vi "Sleep Until Future Time.vi"(7 "FTE Limits (ns)":T1={"Maximum"=200000000, "Minimum"=20000} {"Maximum" format="%.0e"; "Minimum" format="%.0e"}, 8 "error in (no error)":errorcluster, 10 "Wake Time":u64, 11 "ClockID":u16) -> (0 "error out":errorcluster)   [LabVIEW 2021, in "CIFClocks.lvlib"]
uses:
  CIFClocks.lvlib
  Typedef/Future Time Event Limits.ctl
  Typedef/Errors.ctl
  Time Conversion/LabVIEW Time to UTC Time.vi
  CIFCore/CIFCoreCommon/CIFCoreCommon.lvlib
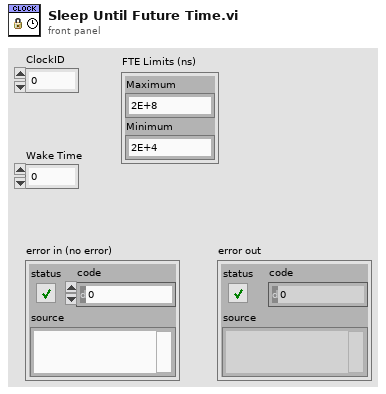
[diagram p1: front panel]
types:
  T1 = typedef "CIFClocks.lvlib/Future Time Event Limits.ctl" = cluster{"Maximum":u64, "Minimum":u64}
  T2 = typedef "CIFCoreCommon.lvlib/Errors.ctl" = enum16{"Invalid Clock ID", "Long Sleep", "gRPC Server Not Found", "Config Parse", "Timestamp Wrap", "Delayed Execution"}
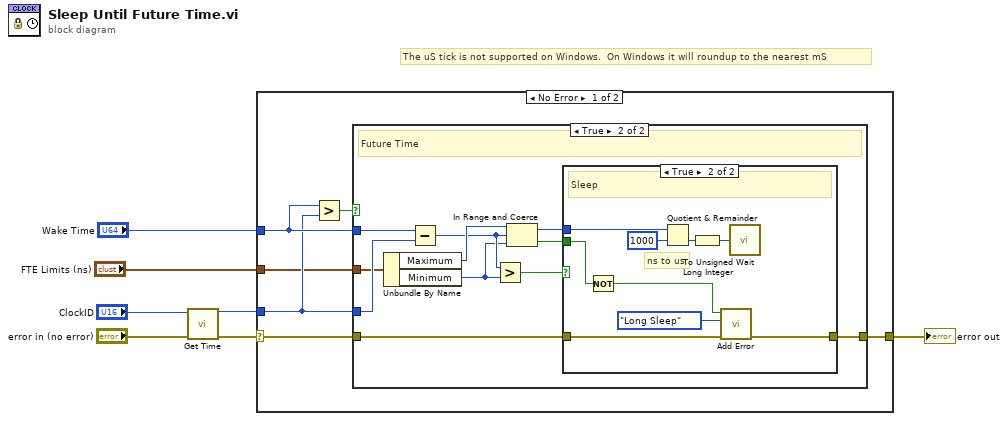
[diagram p0: block diagram]
diagram:
  # "The uS tick is not supported on Windows.  On Windows it will roundup to the nearest mS"
  n1 = call "Get Time.vi"("error in (no error)"="error in (no error)", "ClockID"="ClockID") -> ("error out"=w3:errorcluster, "Time (ns)"=w4:u64)  [unwired: 7 in, 1 out]
  n2 = case shown="No Error" w3 {
    selector: w3 -> [w9 w36]
    tunnel: "Wake Time" -> [w13 _]
    tunnel: w4 -> [w12 _]
    tunnel: [w8 w36] -> w2
    tunnel: "FTE Limits (ns)" -> [w10 _]
    frame No Error {
      n3 = Greater?(x=w13, y=w12) -> (0:w11:bool)
      n4 = case shown="True" w11 {
        tunnel: w13 -> [_ w25]
        tunnel: w12 -> [_ w24]
        tunnel: w10 -> [_ w23]
        tunnel: w9 -> [w14 w20]
        tunnel: [w14 w19] -> w8
        frame False {
          # "Past time, no sleep"
        }
        frame True {
          # "Future Time"
          n5 = Unbundle By Name(w23) -> ("Maximum"=w22:u64, "Minimum"=w17:u64)
          n6 = Subtract(x=w25, y=w24) -> (x-y=w18:u64)
          n7 = Greater?(x=w18, y=w17) -> (0:w16:bool)
          n8 = In Range and Coerce(upper limit=w22, x=w18, lower limit=w17) -> (coerced(x)=w21:u64, In Range?=w15:bool)
          n9 = case shown="True" w16 {
            tunnel: w21 -> [_ w32]
            tunnel: w20 -> [w26 w31]
            tunnel: [w26 w30] -> w19
            tunnel: w15 -> [_ w29]
            frame False {
              # "Sleep less than minimum"
            }
            frame True {
              # "ns to us"
              # "Sleep"
              n10 = Not(x=w29) -> (.not. x?=w28:bool)
              n11 = Quotient & Remainder(x=w32, y=u64 1000) -> (floor(x/y)=w34:u64)  [unwired: 1 out]
              n12 = To Unsigned Long Integer(number=w34) -> (unsigned 32bit integer=w33:u32)
              n13 = call "Add Error.vi"("error in (no error)"=w31, "Error"=Errors."Long Sleep", "Insert Error"=w28) -> ("error out"=w30:errorcluster)  [unwired: 8 in]
              n14 = call "Wait"("Count(uSec)"=w33) -> ()  [unwired: 1 out]
            }
          }
        }
      }
    }
    frame Error {
    }
  }
  "error out" <- w2
